vi "SL_ValueDialog.vi"(8 "type":string, 10 "Value":string, 11 "Title":string) -> (1 "replace?":bool, 2 "Value out":string)   [LabVIEW 2019]
panel:
  in  "Boolean":bool
  in  "Numeric":dbl
  in  "Cancel Button":bool
  in  "OK Button":bool
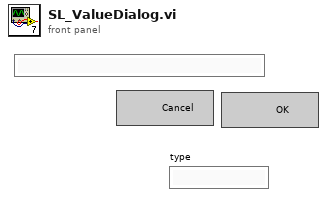
[diagram p1: front panel]
types:
  T1 = enum8{"Enabled", "Disabled", "Disabled and Grayed Out"}
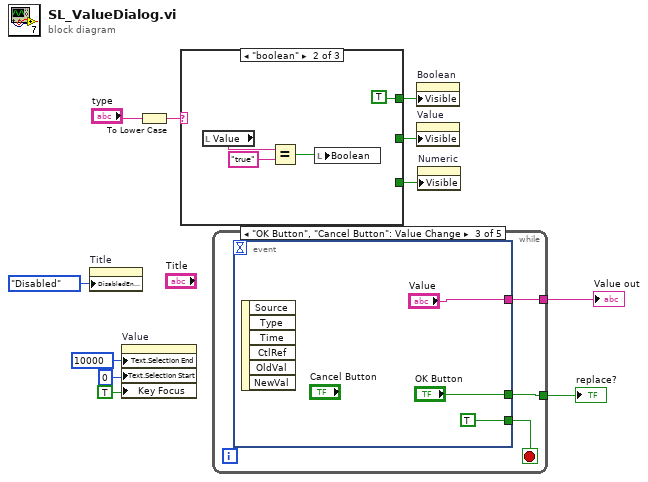
[diagram p0: block diagram]
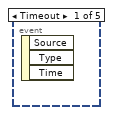
[diagram p2: hidden frame]
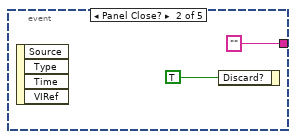
[diagram p3: hidden frame]
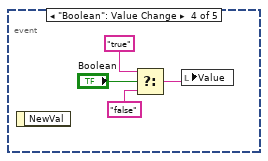
[diagram p4: hidden frame]
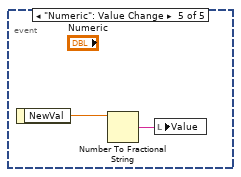
[diagram p5: hidden frame]
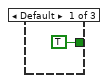
[diagram p6: hidden frame]
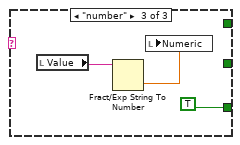
[diagram p7: hidden frame]
diagram:
  n1 = property on="Title" class="Str"("DisabledEnum"=T1."Disabled" ("Disabled")) -> ()  [unwired: 2 in, 2 out]
  n2 = property on="Value" class="Str"("Text.Selection End"=u32 10000 ("Text.Selection:End"), "Text.Selection Start"=u32 0 ("Text.Selection:Start"), "Key Focus"=TRUE) -> ()  [unwired: 2 in, 2 out]
  n3 = To Lower Case(string="type") -> (all lower case string=w4:string)
  n4 = case shown="\"boolean\"" w4 {
    tunnel: [_ TRUE _] -> w3
    tunnel: [_ _ TRUE] -> w2
    tunnel: [TRUE _ _] -> w1
    frame Default {
    }
    frame "boolean" {
      n5 = local read "Value"() -> (w15:string)
      n6 = Equal?(x=w15, y="true") -> (x = y?=w13:bool)
      n7 = local write "Boolean"(w13) -> ()
    }
    frame "number" {
      n8 = local read "Value"() -> (w18:string)
      n9 = Fract/Exp String To Number(string=w18) -> (number=w17:dbl)  [unwired: 3 in, 1 out]
      n10 = local write "Numeric"(w17) -> ()
    }
  }
  n11 = while {
    tunnel: [w22] -> w10
    tunnel: [w21] -> w9
    stop <- w20 stop-if-true
    n12 = event shown="[2] \"OK Button\", \"Cancel Button\": Value Change" {
      selector: _ -> [_ _ _ _ _]
      dyn-events: _ -> [_ _ _ _ _]
      timeout: _ -> [_ _ _ _ _]
      tunnel: [_ _ "OK Button" _ _] -> w22
      tunnel: [_ "" ("Value") "Value" _ _] -> w21
      tunnel: [_ _ TRUE _ _] -> w20
      event Timeout {
        n13 = event-data() -> ()  [unwired: 1 in, 3 out]
      }
      event Panel Close? {
        n14 = event-data() -> ()  [unwired: 1 in, 4 out]
        n15 = event-data("Discard?"=TRUE) -> ()  [unwired: 1 in, 1 out]
      }
      event "OK Button", "Cancel Button": Value Change {
        n16 = event-data() -> ()  [unwired: 1 in, 6 out]
      }
      event "Boolean": Value Change {
        n17 = event-data() -> ()  [unwired: 1 in, 1 out]
        n18 = Select(t="true", s="Boolean", f="false") -> (s? t:f=w30:string)
        n19 = local write "Value"(w30) -> ()
      }
      event "Numeric": Value Change {
        n20 = event-data() -> ("NewVal"=w33:dbl)  [unwired: 1 in]
        n21 = Number To Fractional String(number=w33) -> (F-format string=w32:string)  [unwired: 3 in]
        n22 = local write "Value"(w32) -> ()
      }
    }
  }
  "Value out" <- w9
  "replace?" <- w10
  n23 = property on="Boolean" class="Bool (strict)"("Visible"=w3) -> ()  [unwired: 2 in, 2 out]
  n24 = property on="Value" class="Str"("Visible"=w1) -> ()  [unwired: 2 in, 2 out]
  n25 = property on="Numeric" class="DigNum (strict)"("Visible"=w2) -> ()  [unwired: 2 in, 2 out]
